vi "PH_Beamline.PC _EvacuatedState.vi"(0 "i ref in":refnum<vi>, 2 "Value":i32, 3 "Service Name":string="N/A", 4 "no link":bool, 5 "error IO":errorcluster) -> (14 "i ref out":refnum<vi>, 19 "error out":errorcluster)   [LabVIEW 2014, in "PH_Beamline.lvlib"]
doc: "This VI is the Proc Case \"_Evacuated State\"."
uses:
  PH_Beamline.lvlib
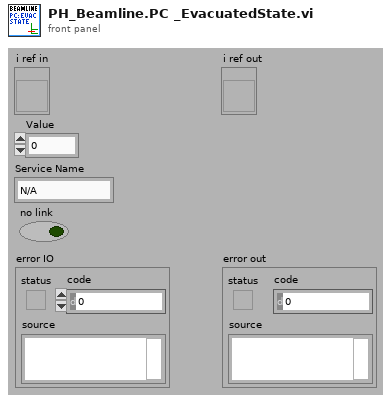
[diagram p1: front panel]
types:
  T1 = typedef "PH_Beamline.lvlib/PH_Beamline.i attribute.ctl" = cluster{"GUI Refs":cluster{"PA ok":refnum<vi>, "MA ok":refnum<vi>, "fs FE ok":refnum<vi>, "ns FE ok":refnum<vi>, "PA ED ok":refnum<vi>, "MAS ok":refnum<vi>, "Booster ok":refnum<vi>, "Mirrortower ok":refnum<vi>, "In.-Box ok":refnum<vi>, "Compressor ok":refnum<vi>, "Experiment LB ok":refnum<vi>, "Experiment LL ok":refnum<vi>, "PHELIX_Beckhoff_Watchdog":refnum<vi>, "Shutters closed":refnum<vi>, "uOPA ok":refnum<vi>, "Vacuum no shotcond Comp LB":refnum<vi>}, "Refs BL MA":refnum<vi>[], "Refs BL MA-IB":refnum<vi>[], "Refs BL fs":refnum<vi>[], "Refs BL PA ED":refnum<vi>[], "Refs BL MAS":refnum<vi>[], "Refs BL Boo":refnum<vi>[], "Refs BL ns":refnum<vi>[], "Refs BL Mirrortower":refnum<vi>[], "Refs BL Compressor":refnum<vi>[], "Refs BL Exp LB":refnum<vi>[], "Radiation Safety":cluster{"Exp Laserbay":cluster{"Ref Op Mode":refnum<vi>, "Ref Laserbay evacuated":refnum<vi>, "Tagname LB evacuated":string, "Shot Mode":T2, "Laserbay evacuated?":i32, "Tagname HV room locked":string, "HV room locked?":i32, "Ref HV room locked":refnum<vi>, "Tagname bridged?":string, "Ref Bridge":refnum<vi>, "I<1E18W/cm²":bool}, "Exp Laserlab":cluster{"Ref Op Mode":refnum<vi>, "Ref Laserlab evacuated":refnum<vi>, "Tagname LL evacuated":string, "Shot Mode":T2, "Laserlab evacuated?":i32, "Tagname bridged?":string, "Ref Bridge":refnum<vi>, "I<1E18W/cm²":bool}}, "Refs BL LL":refnum<vi>[], "PP Igni Heating GUI Refs":refnum<vi>[], "PP Igni Heating Tagnames ":string[], "Refs BL PA":cluster{"undelayed Line before Shutter":refnum<vi>[], "undelayed Line after Shutter":refnum<vi>[], "before Bypass":refnum<vi>[], "delayed Line before Shutter":refnum<vi>[], "delayed Line after Shutter":refnum<vi>[], "before Shutter Input":refnum<vi>[], "after Shutter Input":refnum<vi>[], "Bypass":refnum<vi>[], "before Shutter Exit":refnum<vi>[], "after Shutter Exit":refnum<vi>[], "to MA":refnum<vi>[], "to Lab":refnum<vi>[]}, "BL":cluster{"YLF_BL_Status":i32, "fs_BL_Status":i32, "fs_YLF_BL_Status":i32, "ns_BL_Status":i32, "PA_Input_BL_Status":i32, "PA_UnDelay_BL_Status":i32, "PA_Delay_BL_Status":i32, "PA_BL_Status":i32, "PA_Bypass_BL_Status":i32, "PA_Exit_BL_Status":i32, "PA_LL_BL_Status":i32, "LL_BL_Status":i32, "PA_MA_BL_Status":i32, "MA_Exit_BL_Status":i32, "MA_Z6_BL_Status":i32, "Z6_BL_Status":i32, "MA_LB_BL_Status":i32, "LB_TB2_BL_Status":i32, "PA_before_Bypass_BL_Status":i32, "LB_TB3_BL_Status":i32}, "State Subsystems":cluster{"PA":bool, "MA":bool, "ns FE":bool, "fs FE":bool, "PA ED":bool, "In.-Box":bool, "MAS":bool, "Booster":bool, "Mirrortower":bool, "Compressor":bool, "Experiment LB":bool, "Experiment LL":bool, "uOPA":bool}, "Status Subscriber Information":T3, "Refs BL uOPA":refnum<vi>[], "PA_Input_2_Beam_6PWpGUI not linked?":bool, "PA_Input_Delay_6PGUI not linked?":bool, "Settings":T6}
  T2 = typedef "PH_Beamline.lvlib/PH_Beamline.Operation Mode.ctl" = i32
  T3 = typedef "PH_Beamline.lvlib/PH_Beamline.Status Subscriber Information.ctl" = cluster{"fs Swich YLF":T4, "fs Exit Shutter":T4, "ns Exit Shutter":T4, "PA Input Shutter":T4, "PA PC WP":T4, "PA PC WP 2":T4, "PA Bypass In":T4, "PA Bypass Out":T4, "PA CH 1":T4, "PA delayed":T4, "PA non delayed":T4, "PA Exit Shutter":T4, "PA Switch Lab":T4, "PA Bridge CH Input MA":T4, "MA Diffusor IB":T4, "MA IB Ready":T4, "MA CH 1":T4, "MA CH 2":T4, "MA CH 3":T4, "MA CH 4":T4, "MA Shutter Align Cam":T4, "MA Position MM5":T4, "Calorimeter Switch":T4, "BL Z6 CH 9":T4, "BL Z6 Beamdump":T4, "BL Z6 Shutter":T4, "COS Sensitivity Switch":T4, "Exp LB Shutter":T4, "Exp LB TB 2":T4, "Exp LB TB 3":T4, "PA LL Input CH":T4, "PA LL Output CH":T4, "LL Comp Input Shutter":T4, "LL Comp Output Shutter":T4, "LL Comp FF Shutter":T4, "Exp LL Shutter":T4, "MA IM In IB":T4, "MA IM Out IB":T4, "MA DB In IB":T4, "MA DB Out IB":T4, "Exp LB Shutter Interlock":T4, "Exp LL Shutter Interlock":T4, "MM1 Force Sensor":T4}
  T4 = typedef "PH_BL-Master.lvlib/PH_BL-Master.Status Subscriber Information.ctl" = cluster{"Index of element":i32, "Attributeset":T5}
  T5 = typedef "PH_BL-Master.lvlib/PH_BL-Master.Attribute Set.ctl" = enum16{"Boolean Status Service Subscriber", "Picture Status Service Subscriber"}
  T6 = typedef "PH_Beamline_Chief.lvlib/PH_Beamline_Chief.Settings.ctl" = cluster{"PA Doublepass Mode":bool, "Compressor Vaccuum LB not relevant":bool, "Windowshutter TB2 not relevant":bool, "Windowshutter TB3 not relevant":bool}
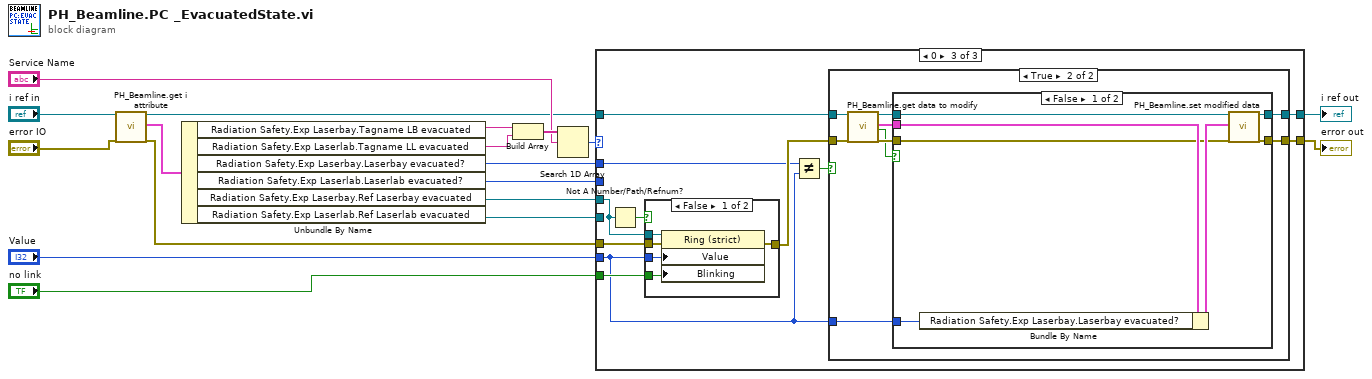
[diagram p0: block diagram]
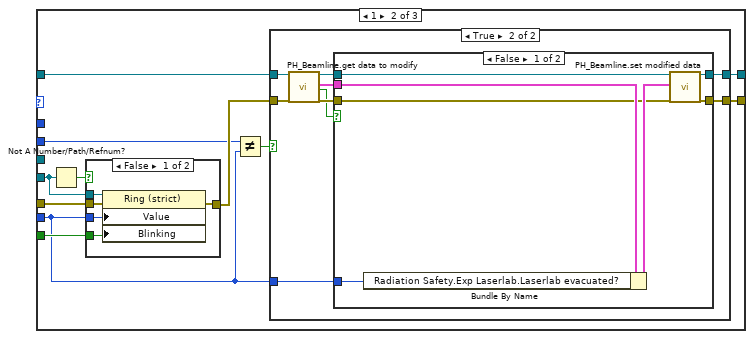
[diagram p3: hidden frame]
diagram:
  n1 = call "PH_Beamline.get i attribute.vi"("i ref in"="i ref in", "error in (no error)"="error IO") -> ("i ref out"=w7:refnum<vi>, "i attribute"=w18:T1, "error out"=w17:errorcluster)  [unwired: 15 in]
  n2 = Unbundle By Name(w18) -> ("Radiation Safety.Exp Laserbay.Tagname LB evacuated"=w15:string, "Radiation Safety.Exp Laserlab.Tagname LL evacuated"=w16:string, "Radiation Safety.Exp Laserbay.Laserbay evacuated?"=w2:i32, "Radiation Safety.Exp Laserlab.Laserlab evacuated?"=w3:i32, "Radiation Safety.Exp Laserbay.Ref Laserbay evacuated"=w1:refnum<vi>, "Radiation Safety.Exp Laserlab.Ref Laserlab evacuated"=w4:refnum<vi>)
  n3 = Build Array(w15, w16) -> (w14:string[])
  n4 = Search 1D Array(1D array=w14, element="Service Name") -> (index of element=w13:i32)  [unwired: 1 in]
  n5 = case shown="0" w13 {
    tunnel: w17 -> [w20 w31 w68]
    tunnel: "Value" -> [_ w23 w60]
    tunnel: "no link" -> [_ w30 w67]
    tunnel: w7 -> [w19 w28 w65]
    tunnel: [w19 w27 w64] -> w6
    tunnel: [w20 w26 w63] -> w5
    tunnel: w4 -> [_ w22 _]
    tunnel: w3 -> [_ w21 _]
    tunnel: w2 -> [_ _ w59]
    tunnel: w1 -> [_ _ w58]
    frame Default {
    }
    frame 1 {
      n6 = Not A Number/Path/Refnum?(number/path/refnum=w22) -> (NaN/Path/Refnum?=w29:bool)
      n7 = case shown="False" w29 {
        tunnel: w31 -> [w56 w57]
        tunnel: [w55 w57] -> w25
        tunnel: w22 -> [w54 _]
        tunnel: w23 -> [w53 _]
        tunnel: w30 -> [w52 _]
        frame False {
          n8 = property class="Ring (strict)"(reference=w54, error in=w56, "Value"=w53, "Blinking"=w52) -> (error out=w55:errorcluster)  [unwired: 1 out]
        }
        frame True {
        }
      }
      n9 = Not Equal?(x=w21, y=w23) -> (x != y?=w24:bool)
      n10 = case shown="True" w24 {
        tunnel: w28 -> [w33 w38]
        tunnel: [w33 w37] -> w27
        tunnel: [w32 w36] -> w26
        tunnel: w25 -> [w32 w35]
        tunnel: w23 -> [_ w34]
        frame False {
        }
        frame True {
          n11 = call "PH_Beamline.get data to modify.vi"("i ref in"=w38, "error in (no error)"=w35) -> ("i ref out"=w41:refnum<vi>, "i attribute"=w39:T1, "timed out"=w40:bool, "error out"=w42:errorcluster)  [unwired: 14 in]
          n12 = case shown="False" w40 {
            tunnel: w42 -> [w43 w50]
            tunnel: w41 -> [w49 w51]
            tunnel: [w48 w51] -> w37
            tunnel: [w47 w50] -> w36
            tunnel: w39 -> [w45 _]
            tunnel: w34 -> [w44 _]
            frame False {
              n13 = Bundle By Name(cluster=w45, "Radiation Safety.Exp Laserlab.Laserlab evacuated?"=w44) -> (w46:T1)
              n14 = call "PH_Beamline.set modified data.vi"("i ref in"=w49, "i attribute"=w46, "error in (no error)"=w43) -> ("i ref out"=w48:refnum<vi>, "error out"=w47:errorcluster)  [unwired: 15 in]
            }
            frame True {
            }
          }
        }
      }
    }
    frame 0 {
      n15 = Not A Number/Path/Refnum?(number/path/refnum=w58) -> (NaN/Path/Refnum?=w66:bool)
      n16 = case shown="False" w66 {
        tunnel: w68 -> [w93 w94]
        tunnel: [w92 w94] -> w62
        tunnel: w58 -> [w91 _]
        tunnel: w60 -> [w90 _]
        tunnel: w67 -> [w89 _]
        frame False {
          n17 = property class="Ring (strict)"(reference=w91, error in=w93, "Value"=w90, "Blinking"=w89) -> (error out=w92:errorcluster)  [unwired: 1 out]
        }
        frame True {
        }
      }
      n18 = Not Equal?(x=w59, y=w60) -> (x != y?=w61:bool)
      n19 = case shown="True" w61 {
        tunnel: w65 -> [w70 w75]
        tunnel: [w70 w74] -> w64
        tunnel: [w69 w73] -> w63
        tunnel: w62 -> [w69 w72]
        tunnel: w60 -> [_ w71]
        frame False {
        }
        frame True {
          n20 = call "PH_Beamline.get data to modify.vi"("i ref in"=w75, "error in (no error)"=w72) -> ("i ref out"=w78:refnum<vi>, "i attribute"=w76:T1, "timed out"=w77:bool, "error out"=w79:errorcluster)  [unwired: 14 in]
          n21 = case shown="False" w77 {
            tunnel: w79 -> [w80 w87]
            tunnel: w78 -> [w86 w88]
            tunnel: [w85 w88] -> w74
            tunnel: [w84 w87] -> w73
            tunnel: w76 -> [w82 _]
            tunnel: w71 -> [w81 _]
            frame False {
              n22 = Bundle By Name(cluster=w82, "Radiation Safety.Exp Laserbay.Laserbay evacuated?"=w81) -> (w83:T1)
              n23 = call "PH_Beamline.set modified data.vi"("i ref in"=w86, "i attribute"=w83, "error in (no error)"=w80) -> ("i ref out"=w85:refnum<vi>, "error out"=w84:errorcluster)  [unwired: 15 in]
            }
            frame True {
            }
          }
        }
      }
    }
  }
  "error out" <- w5
  "i ref out" <- w6
